vi "GUILoop.vi"(8 "error in (no error)":errorcluster, 10 "ctrls":T2, 11 "Queue cluster":T1) -> ()   [LabVIEW 2017]
uses:
  controls_main.ctl
  QueueCluster.ctl
  EventQueueCluster.ctl
  EventMessage.ctl
  MeasureQueue.ctl
  MeasureMessage.ctl
  HardwareQueueCluster.ctl
  hardwareMessage.ctl
  GUIQueueCluster.ctl
  GUIMessage.ctl
  SaveQueueCluster.ctl
  SaveMessage.ctl
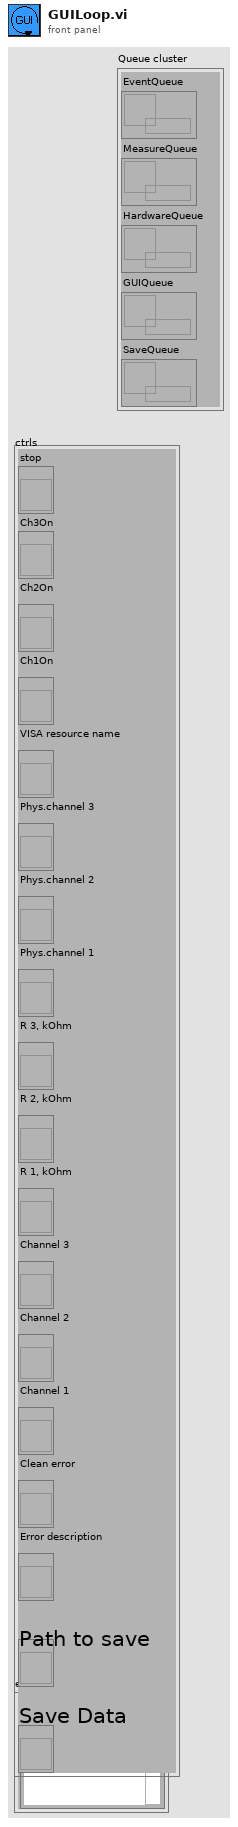
[diagram p1: front panel]
types:
  T1 = typedef "QueueCluster.ctl" = cluster{"EventQueue":refnum<queue>, "MeasureQueue":refnum<queue>, "HardwareQueue":refnum<queue>, "GUIQueue":refnum<queue>, "SaveQueue":refnum<queue>}
  T2 = typedef "controls_main.ctl" = cluster{"stop":refnum<vi>, "Ch3On":refnum<vi>, "Ch2On":refnum<vi>, "Ch1On":refnum<vi>, "VISA resource name":refnum<vi>, "Phys.channel 3":refnum<vi>, "Phys.channel 2":refnum<vi>, "Phys.channel 1":refnum<vi>, "R 3, kOhm":refnum<vi>, "R 2, kOhm":refnum<vi>, "R 1, kOhm":refnum<vi>, "Channel 3":refnum<vi>, "Channel 2":refnum<vi>, "Channel 1":refnum<vi>, "Clean error":refnum<vi>, "Error description":refnum<vi>, "Path to save":refnum<vi>, "Save Data":refnum<vi>}
  T3 = enum8{"Enabled", "Disabled", "Disabled and Grayed Out"}
  T4 = typedef "GUIQueueCluster.ctl" = cluster{"GUIMessage":T5, "NumericValue":dbl, "String":string}
  T5 = typedef "GUIMessage.ctl" = enum16{"StopSave", "Channel1Value", "Channel2Value", "Channel3Value", "ErrorSource", "CleanError", "StartChannel1", "StartChannel2", "StartChannel3", "StopChannel1", "StopChannel2", "StopChannel3", "Halt"}
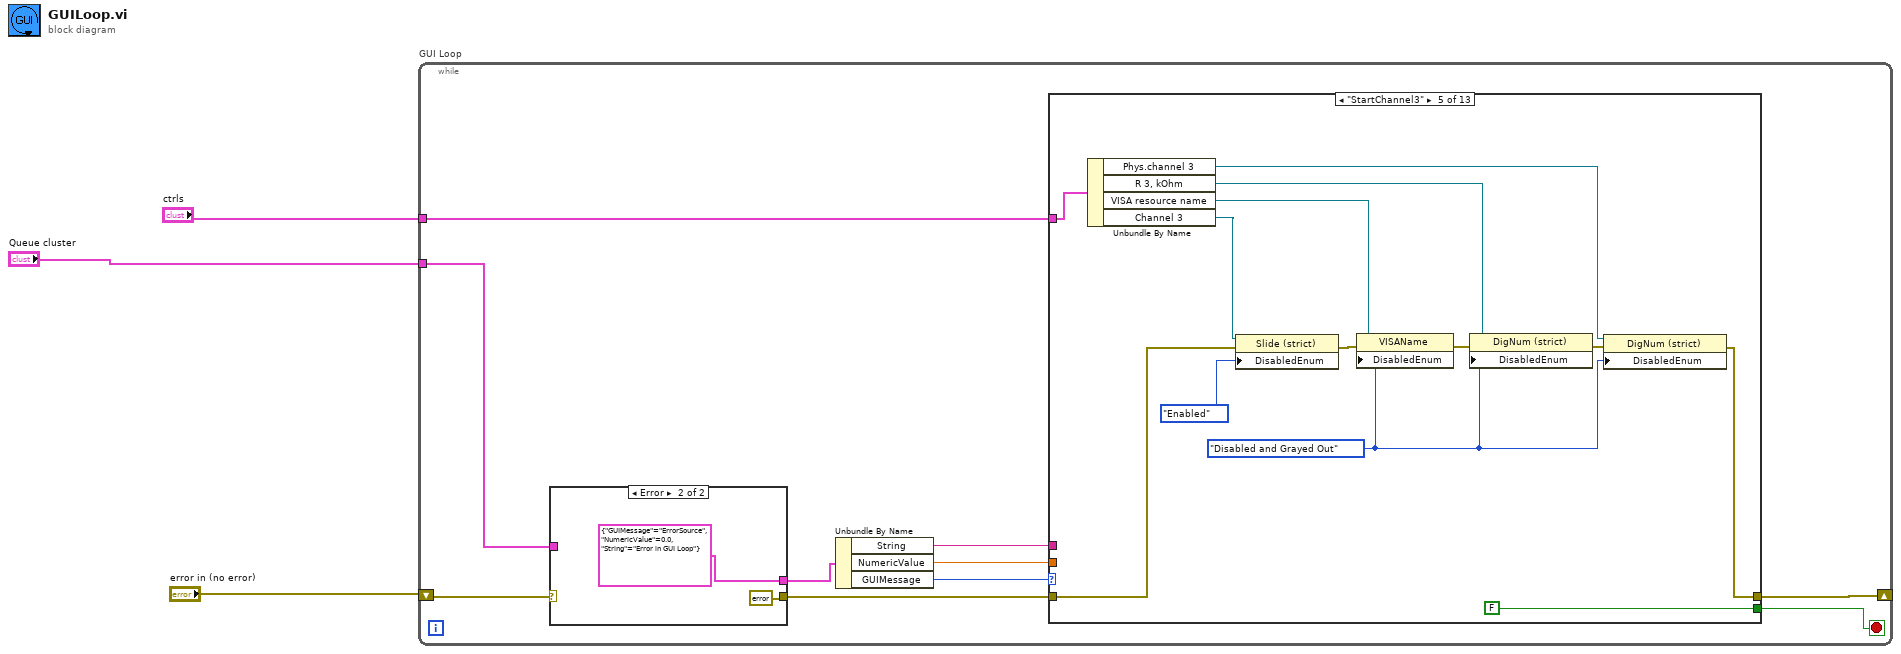
[diagram p0: block diagram]
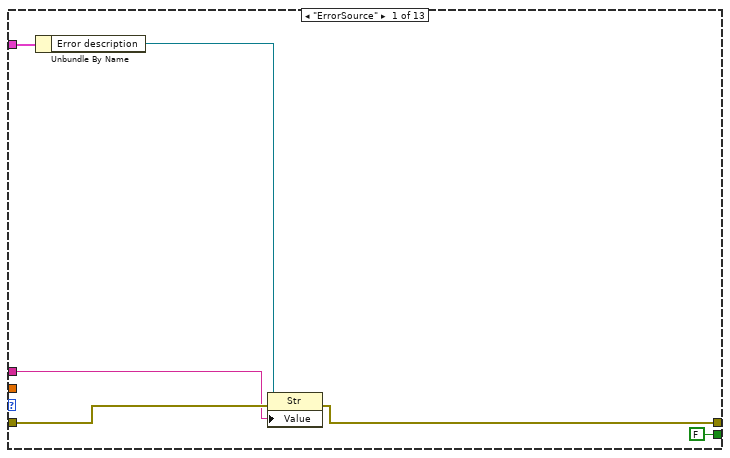
[diagram p2: hidden frame]
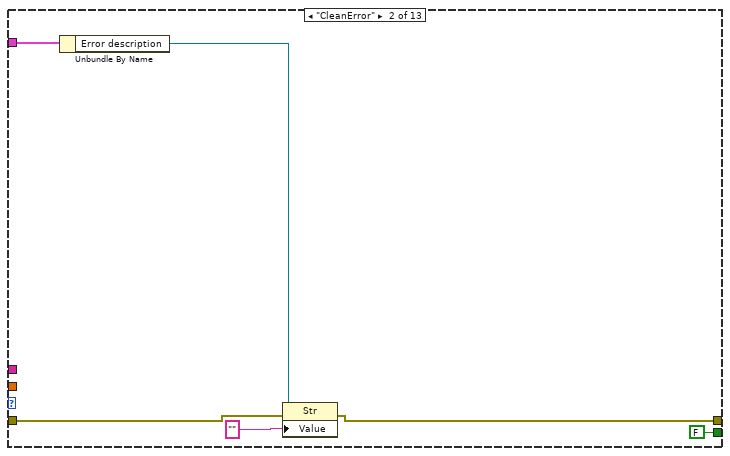
[diagram p3: hidden frame]
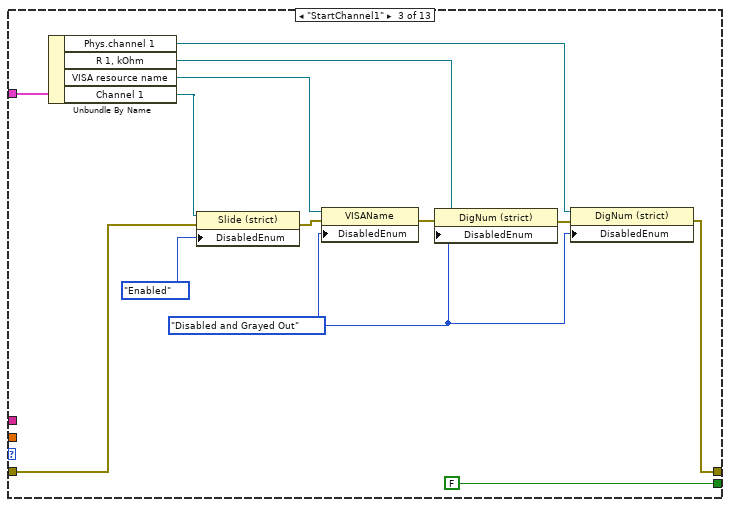
[diagram p4: hidden frame]
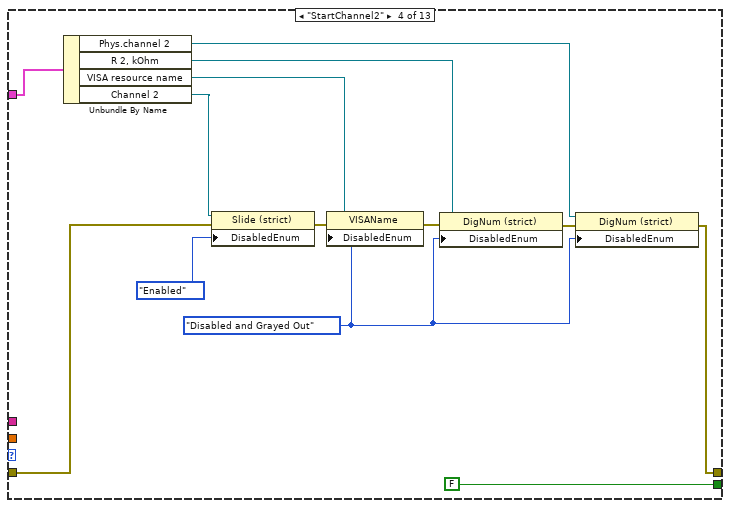
[diagram p5: hidden frame]
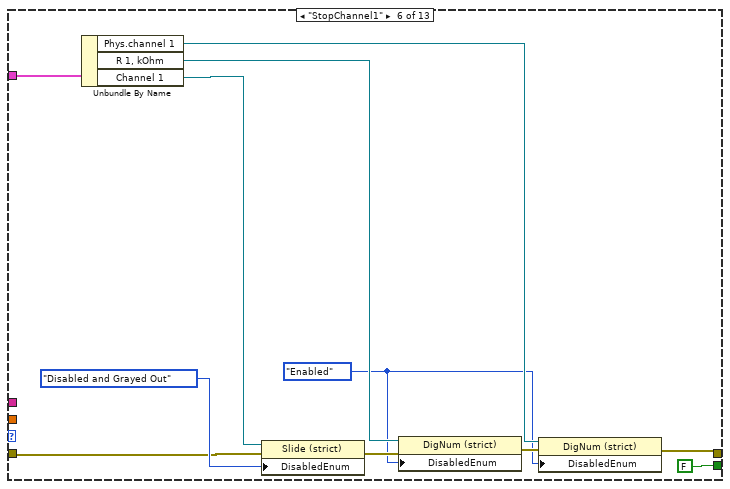
[diagram p6: hidden frame]
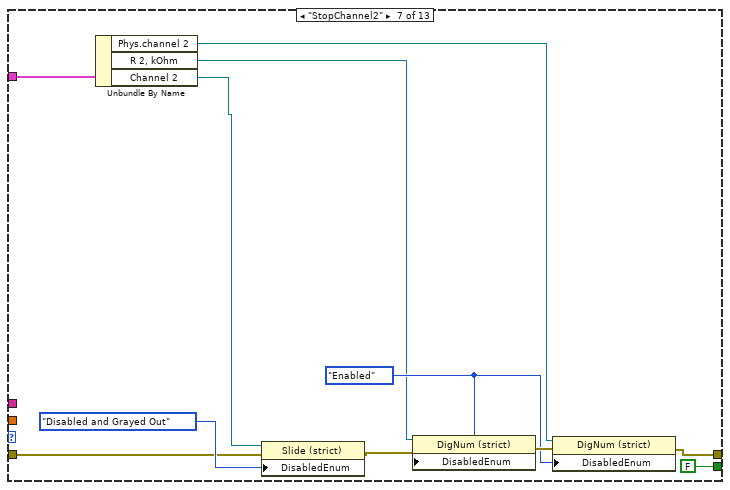
[diagram p7: hidden frame]
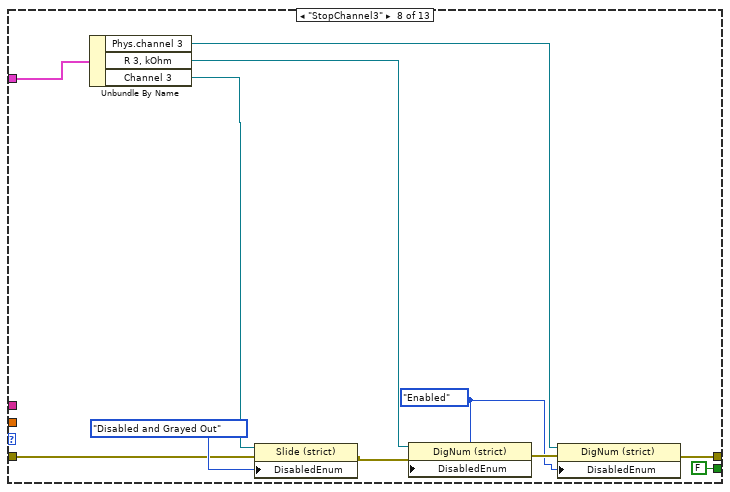
[diagram p8: hidden frame]
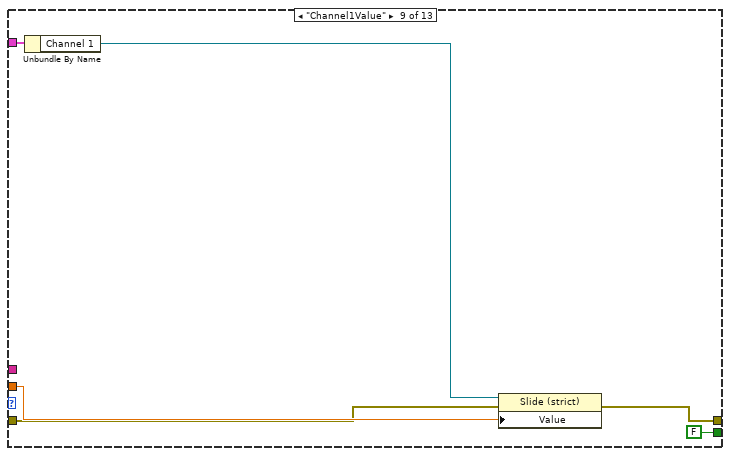
[diagram p9: hidden frame]
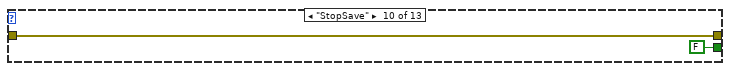
[diagram p10: hidden frame]
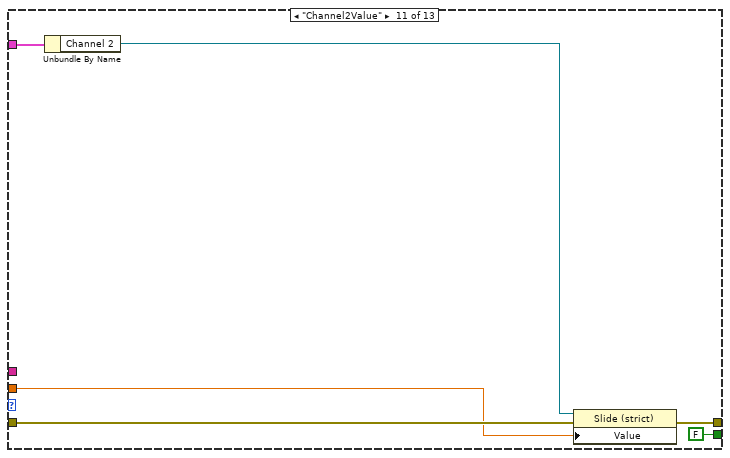
[diagram p11: hidden frame]
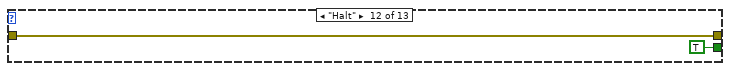
[diagram p12: hidden frame]
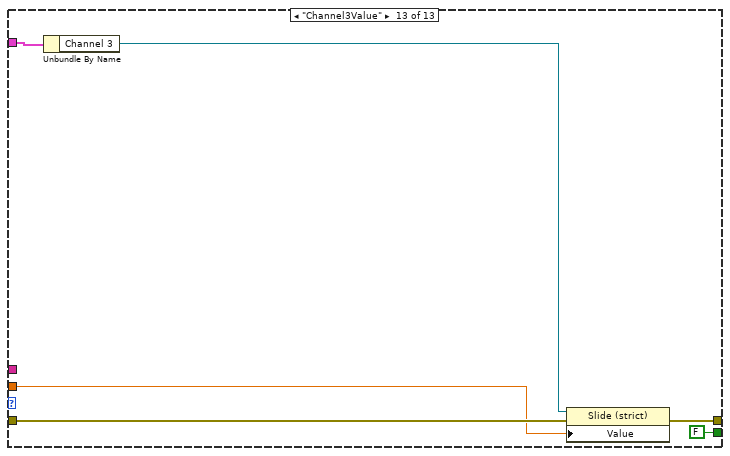
[diagram p13: hidden frame]
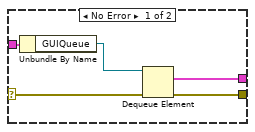
[diagram p14: hidden frame]
diagram:
  n1 = while "GUI Loop" {
    tunnel: "ctrls" -> [w8]
    tunnel: "Queue cluster" -> [w12]
    shift-right: [w6] -> _
    shift-left: "error in (no error)" -> [w13]
    stop <- w5 stop-if-true
    n2 = case shown="Error" w13 {
      selector: w13 -> [w124 _]
      tunnel: w12 -> [w123 _]
      tunnel: [w121 errorcluster {"status"=FALSE, "code"=0, "source"=""} ("error out")] -> w10
      tunnel: [w120 T4 {"GUIMessage"=enum."ErrorSource", "NumericValue"=0.0, "String"="Error in GUI Loop"} ("GUIQueueCluster")] -> w11
      frame No Error {
        n3 = Unbundle By Name(w123) -> ("GUIQueue"=w122:refnum<queue>)
        n4 = Dequeue Element(queue=w122, error in (no error)=w124) -> (element=w120:T4, error out=w121:errorcluster)  [unwired: 1 in, 2 out]
      }
      frame Error {
      }
    }
    n5 = Unbundle By Name(w11) -> ("String"=w4:string, "NumericValue"=w7:dbl, "GUIMessage"=w9:T5)
    n6 = case shown="\"StartChannel3\"" w9 {
      tunnel: w10 -> [w17 w22 w35 w44 w57 w72 w83 w94 w98 w105 w107 w112 w115]
      tunnel: w8 -> [w19 w25 w36 w43 w56 w73 w84 w95 w103 _ w109 _ w118]
      tunnel: w7 -> [_ _ _ _ _ _ _ _ w99 _ w106 _ w114]
      tunnel: [w15 w21 w26 w39 w52 w66 w79 w90 w101 w105 w108 w112 w117] -> w6
      tunnel: [FALSE FALSE FALSE FALSE FALSE FALSE FALSE FALSE FALSE FALSE FALSE TRUE FALSE] -> w5
      tunnel: w4 -> [w16 _ _ _ _ _ _ _ _ _ _ _ _]
      frame "ErrorSource" {
        n7 = Unbundle By Name(w19) -> ("Error description"=w18:refnum<vi>)
        n8 = property class="Str"(reference=w18, error in=w17, "Value"=w16) -> (error out=w15:errorcluster)  [unwired: 1 out]
      }
      frame "CleanError" {
        n9 = Unbundle By Name(w25) -> ("Error description"=w24:refnum<vi>)
        n10 = property class="Str"(reference=w24, error in=w22, "Value"="") -> (error out=w21:errorcluster)  [unwired: 1 out]
      }
      frame "StartChannel1" {
        w27 = T3."Disabled and Grayed Out" ("Disabled")
        n11 = Unbundle By Name(w36) -> ("Phys.channel 1"=w29:refnum<vi>, "R 1, kOhm"=w31:refnum<vi>, "VISA resource name"=w33:refnum<vi>, "Channel 1"=w37:refnum<vi>)
        n12 = property class="Slide (strict)"(reference=w37, error in=w35, "DisabledEnum"=T3."Enabled" ("Disabled")) -> (error out=w32:errorcluster)  [unwired: 1 out]
        n13 = property class="VISAName"(reference=w33, error in=w32, "DisabledEnum"=w27) -> (error out=w30:errorcluster)  [unwired: 1 out]
        n14 = property class="DigNum (strict)"(reference=w31, error in=w30, "DisabledEnum"=w27) -> (error out=w28:errorcluster)  [unwired: 1 out]
        n15 = property class="DigNum (strict)"(reference=w29, error in=w28, "DisabledEnum"=w27) -> (error out=w26:errorcluster)  [unwired: 1 out]
      }
      frame "StartChannel2" {
        w40 = T3."Disabled and Grayed Out" ("Disabled")
        n16 = Unbundle By Name(w43) -> ("Phys.channel 2"=w42:refnum<vi>, "R 2, kOhm"=w46:refnum<vi>, "VISA resource name"=w48:refnum<vi>, "Channel 2"=w50:refnum<vi>)
        n17 = property class="Slide (strict)"(reference=w50, error in=w44, "DisabledEnum"=T3."Enabled" ("Disabled")) -> (error out=w47:errorcluster)  [unwired: 1 out]
        n18 = property class="VISAName"(reference=w48, error in=w47, "DisabledEnum"=w40) -> (error out=w45:errorcluster)  [unwired: 1 out]
        n19 = property class="DigNum (strict)"(reference=w46, error in=w45, "DisabledEnum"=w40) -> (error out=w41:errorcluster)  [unwired: 1 out]
        n20 = property class="DigNum (strict)"(reference=w42, error in=w41, "DisabledEnum"=w40) -> (error out=w39:errorcluster)  [unwired: 1 out]
      }
      frame "StartChannel3" {
        w53 = T3."Disabled and Grayed Out" ("Disabled")
        n21 = Unbundle By Name(w56) -> ("Phys.channel 3"=w55:refnum<vi>, "R 3, kOhm"=w59:refnum<vi>, "VISA resource name"=w61:refnum<vi>, "Channel 3"=w63:refnum<vi>)
        n22 = property class="Slide (strict)"(reference=w63, error in=w57, "DisabledEnum"=T3."Enabled" ("Disabled")) -> (error out=w60:errorcluster)  [unwired: 1 out]
        n23 = property class="VISAName"(reference=w61, error in=w60, "DisabledEnum"=w53) -> (error out=w58:errorcluster)  [unwired: 1 out]
        n24 = property class="DigNum (strict)"(reference=w59, error in=w58, "DisabledEnum"=w53) -> (error out=w54:errorcluster)  [unwired: 1 out]
        n25 = property class="DigNum (strict)"(reference=w55, error in=w54, "DisabledEnum"=w53) -> (error out=w52:errorcluster)  [unwired: 1 out]
      }
      frame "StopChannel1" {
        w65 = T3."Enabled" ("Disabled")
        n26 = Unbundle By Name(w73) -> ("Phys.channel 1"=w68:refnum<vi>, "R 1, kOhm"=w70:refnum<vi>, "Channel 1"=w75:refnum<vi>)
        n27 = property class="Slide (strict)"(reference=w75, error in=w72, "DisabledEnum"=T3."Disabled and Grayed Out" ("Disabled")) -> (error out=w69:errorcluster)  [unwired: 1 out]
        n28 = property class="DigNum (strict)"(reference=w70, error in=w69, "DisabledEnum"=w65) -> (error out=w67:errorcluster)  [unwired: 1 out]
        n29 = property class="DigNum (strict)"(reference=w68, error in=w67, "DisabledEnum"=w65) -> (error out=w66:errorcluster)  [unwired: 1 out]
      }
      frame "StopChannel2" {
        w78 = T3."Enabled" ("Disabled")
        n30 = Unbundle By Name(w84) -> ("Phys.channel 2"=w76:refnum<vi>, "R 2, kOhm"=w77:refnum<vi>, "Channel 2"=w86:refnum<vi>)
        n31 = property class="Slide (strict)"(reference=w86, error in=w83, "DisabledEnum"=T3."Disabled and Grayed Out" ("Disabled")) -> (error out=w80:errorcluster)  [unwired: 1 out]
        n32 = property class="DigNum (strict)"(reference=w77, error in=w80, "DisabledEnum"=w78) -> (error out=w81:errorcluster)  [unwired: 1 out]
        n33 = property class="DigNum (strict)"(reference=w76, error in=w81, "DisabledEnum"=w78) -> (error out=w79:errorcluster)  [unwired: 1 out]
      }
      frame "StopChannel3" {
        w87 = T3."Enabled" ("Disabled")
        n34 = Unbundle By Name(w95) -> ("Phys.channel 3"=w88:refnum<vi>, "R 3, kOhm"=w89:refnum<vi>, "Channel 3"=w97:refnum<vi>)
        n35 = property class="Slide (strict)"(reference=w97, error in=w94, "DisabledEnum"=T3."Disabled and Grayed Out" ("Disabled")) -> (error out=w91:errorcluster)  [unwired: 1 out]
        n36 = property class="DigNum (strict)"(reference=w89, error in=w91, "DisabledEnum"=w87) -> (error out=w92:errorcluster)  [unwired: 1 out]
        n37 = property class="DigNum (strict)"(reference=w88, error in=w92, "DisabledEnum"=w87) -> (error out=w90:errorcluster)  [unwired: 1 out]
      }
      frame "Channel1Value" {
        n38 = Unbundle By Name(w103) -> ("Channel 1"=w102:refnum<vi>)
        n39 = property class="Slide (strict)"(reference=w102, error in=w98, "Value"=w99) -> (error out=w101:errorcluster)  [unwired: 1 out]
      }
      frame "StopSave" {
      }
      frame "Channel2Value" {
        n40 = Unbundle By Name(w109) -> ("Channel 2"=w110:refnum<vi>)
        n41 = property class="Slide (strict)"(reference=w110, error in=w107, "Value"=w106) -> (error out=w108:errorcluster)  [unwired: 1 out]
      }
      frame "Halt" {
      }
      frame "Channel3Value" {
        n42 = Unbundle By Name(w118) -> ("Channel 3"=w119:refnum<vi>)
        n43 = property class="Slide (strict)"(reference=w119, error in=w115, "Value"=w114) -> (error out=w117:errorcluster)  [unwired: 1 out]
      }
    }
  }
